vi "Modbus_TCP.vi"() -> ()   [LabVIEW 2024]
uses:
  <vilib>/NI/Modbus Library/API/Wrapper/Create TCP Master.vi
  <vilib>/NI/Modbus Library/API/Master/Modbus Master.lvclass
  <vilib>/NI/Modbus Library/API/Wrapper/API Main.lvlib
panel:
  in  "error in":errorcluster
  in  "number of inputs":u16
  in  "starting address":u16
  in  "stop":bool
  out "read values":u16[](array[numeric])
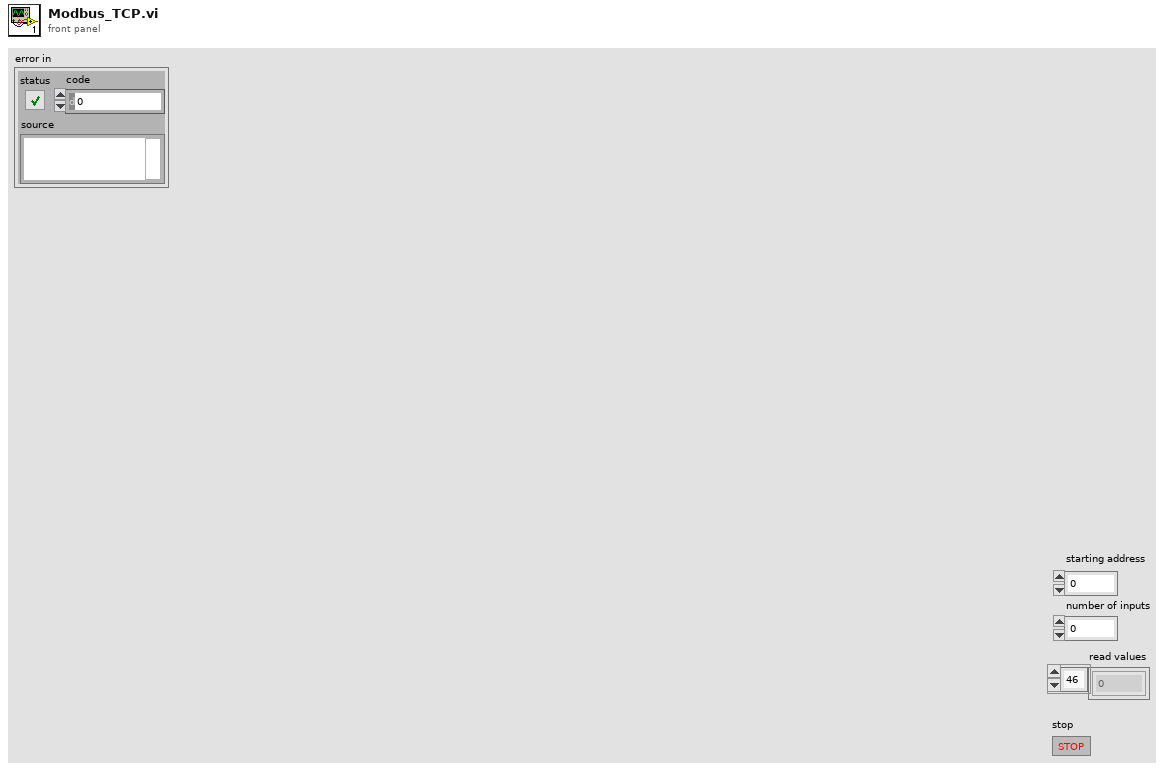
[diagram p1: front panel]
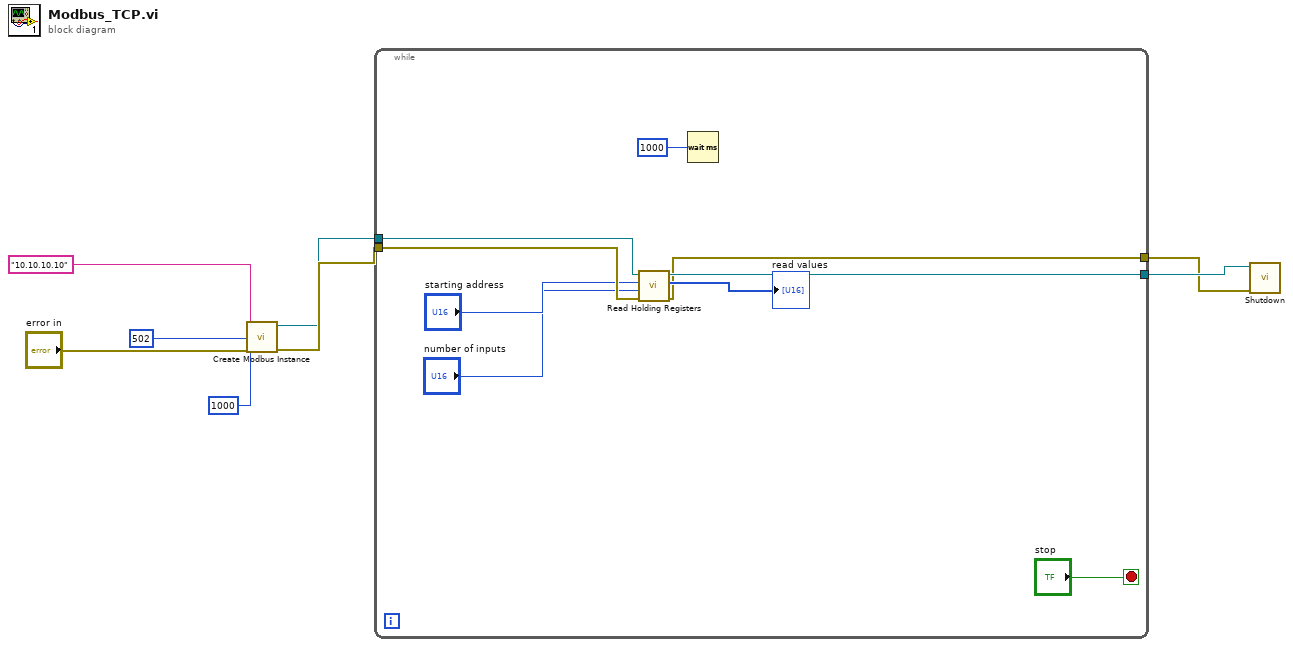
[diagram p0: block diagram]
diagram:
  n1 = call-poly <vilib>:"Create Modbus Instance.vi"("error in"="error in", "connect timeout ms"=1000, "port (502)"=u16 502, "address"="10.10.10.10") -> ("error out"=w8:errorcluster, "TCP master instance"=w7:refnum<class "Modbus Master.lvclass">)  [unwired: 6 in]
  n2 = while {
    tunnel: w7 -> [w14]
    tunnel: w8 -> [w13]
    tunnel: [w10] -> w2
    tunnel: [w9] -> w1
    stop <- "stop" stop-if-true
    n3 = call-dynamic "Read Holding Registers.vi"("error in"=w13, "number of inputs"="number of inputs", "starting address"="starting address", "Modbus master in"=w14) -> ("error out"=w9:errorcluster, "register values"=→"read values":u16[], "Modbus master out"=w10:refnum<class "Modbus Master.lvclass">)  [unwired: 5 in]
    n4 = Wait (ms)(milliseconds to wait=u32 1000) -> ()  [unwired: 1 out]
  }
  n5 = call-dynamic "Shutdown.vi"("error in"=w1, "Modbus master in"=w2) -> ()  [unwired: 9 in, 1 out]
